vi "MRC Smart IO Set Led Length.vi"(8 "error in (no error)":errorcluster, 10 "length":i32, 11 "deviceIndex":i32) -> (0 "error out":errorcluster)   [LabVIEW 2026, in "MrcLib.lvlib"]
doc: "MRC_Status MRC_CALLCONV MRC_SmartIO_SetLedLength(int32_t deviceIndex, int32_t length);"
uses:
  MrcLib.lvlib
  MrcLib.so
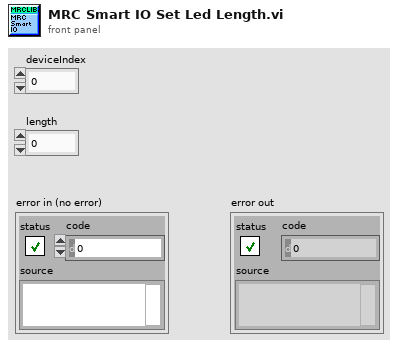
[diagram p1: front panel]
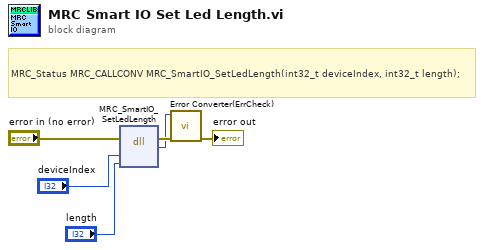
[diagram p0: block diagram]
diagram:
  # "MRC_Status MRC_CALLCONV MRC_SmartIO_SetLedLength(int32_t deviceIndex, int32_t length);"
  n1 = dll-call lib="MrcLib.*" fn="MRC_SmartIO_SetLedLength"(error in="error in (no error)", "deviceIndex"="deviceIndex", "length"="length") -> (error out=w3:errorcluster, w1:i32)  [unwired: 4 in, 1 out]
  n2 = call "Error Converter(ErrCheck).vi"("error in (no error)"=w3, "status"=w1) -> ("error out"=→"error out":errorcluster)  [unwired: 9 in]
